vi "发送数据记录到文档(子VI).vi"(7 "错误输入":errorcluster, 9 "字符串":string="报文记录", 10 "数组":string[](array[string])) -> (0 "错误输出":errorcluster)   [LabVIEW 2022 SP3, in "工况数据上传.lvlib"]
panel:
  out "路径":path
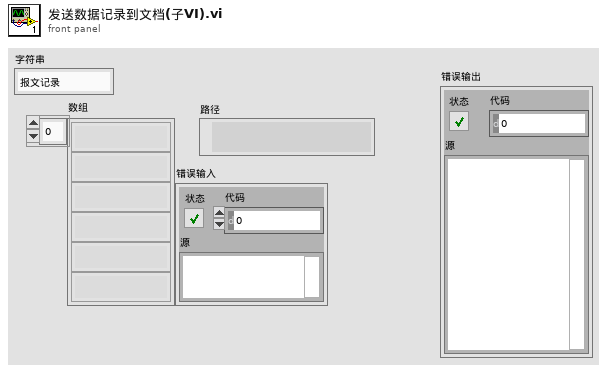
[diagram p1: front panel]
types:
  T1 = typedef "LVDateTimeRec.ctl" = cluster{"秒数的小数部分":dbl, "秒":i32, "分":i32, "时":i32, "日":i32, "月":i32, "年":i32, "天数（周）":i32, "天数（年）":i32, "DST":i32}
  T2 = enum16{"open", "replace", "create", "open or create", "replace or create", "replace or create with confirmation"}
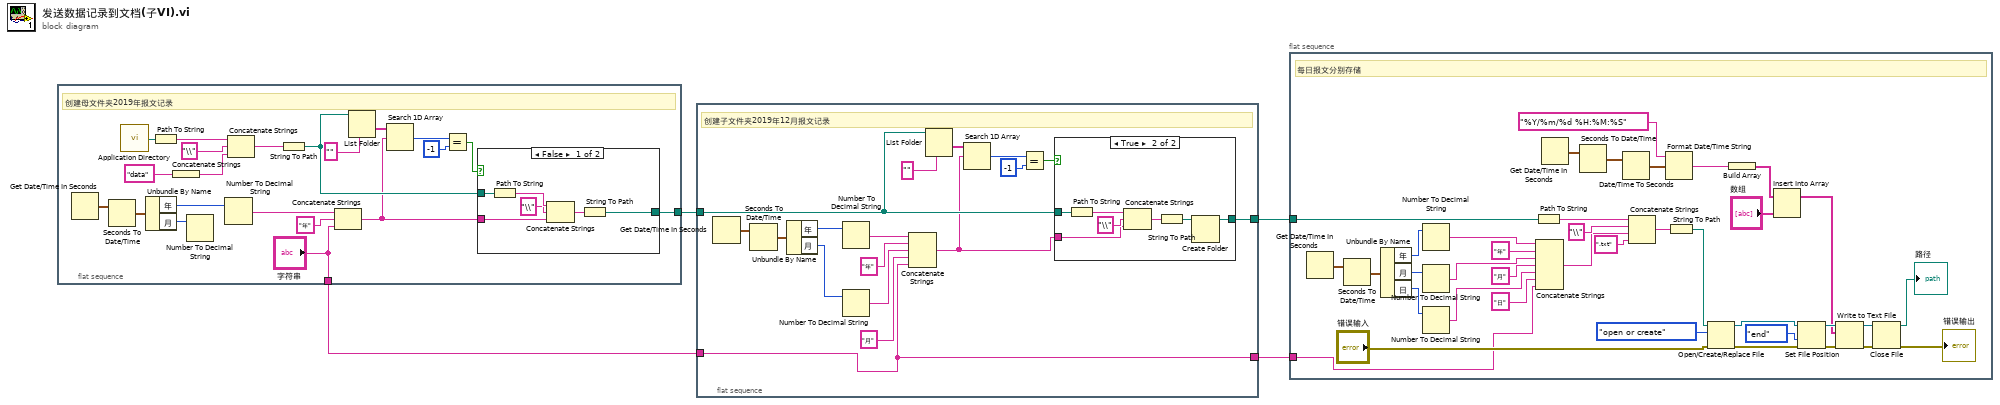
[diagram p0: block diagram]
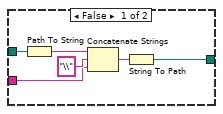
[diagram p2: hidden frame]
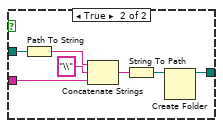
[diagram p3: hidden frame]
diagram:
  n1 = flat-sequence {
    tunnel: [w8] -> w4
    tunnel: ["字符串"] -> w2
    frame #0 {
      # "创建母文件夹2019年报文记录"
      n2 = Get Date/Time In Seconds() -> (seconds since 1Jan1904=w25:timestamp)
      n3 = Seconds To Date/Time(time stamp (now)=w25) -> (date time rec=w24:T1)  [unwired: 1 in]
      n4 = call <vilib>:"Application Directory.vi"() -> ("Application Directory"=w13:path)
      n5 = Unbundle By Name(w24) -> ("年"=w23:i32, "月"=w22:i32)
      n6 = Path To String(path=w13) -> (string=w16:string)
      n7 = Concatenate Strings("data" ("名称或相对路径")) -> (w5:string)
      n8 = Number To Decimal String(number=w22) -> ()  [unwired: 1 in, 1 out]
      n9 = Number To Decimal String(number=w23) -> (decimal integer string=w10:string)  [unwired: 1 in]
      n10 = Concatenate Strings(w16, "\\" ("字符串"), w5) -> (w14:string)
      n11 = String To Path(string=w14) -> (path=w12:path)
      n12 = Concatenate Strings(w10, "年" ("字符串"), "字符串") -> (w9:string)
      n13 = List Folder(path=w12, pattern="" ("类型")) -> (folder names=w17:string[])  [unwired: 2 in, 3 out]
      n14 = Search 1D Array(1D array=w17, element=w9) -> (index of element=w21:i32)  [unwired: 1 in]
      n15 = Equal?(x=w21, y=-1) -> (x = y?=w19:bool)
      n16 = case shown="False" w19 {
        tunnel: w12 -> [w29 w37]
        tunnel: w9 -> [w28 w34]
        tunnel: [w27 w38] -> w8
        frame False {
          n17 = Path To String(path=w29) -> (string=w31:string)
          n18 = Concatenate Strings(w31, "\\" ("字符串"), w28) -> (w26:string)
          n19 = String To Path(string=w26) -> (path=w27:path)
        }
        frame True {
          n20 = Path To String(path=w37) -> (string=w36:string)
          n21 = Concatenate Strings(w36, "\\" ("字符串"), w34) -> (w32:string)
          n22 = String To Path(string=w32) -> (path=w33:path)
          n23 = Create Folder(path (use dialog)=w33) -> (created path=w38:path)  [unwired: 2 in, 2 out]
        }
      }
    }
  }
  n24 = flat-sequence {
    tunnel: w4 -> [w42]
    tunnel: [w40] -> w3
    tunnel: w2 -> [w39]
    tunnel: [w39] -> w1
    frame #0 {
      # "创建子文件夹2019年12月报文记录"
      n25 = Get Date/Time In Seconds() -> (seconds since 1Jan1904=w45:timestamp)
      n26 = Seconds To Date/Time(time stamp (now)=w45) -> (date time rec=w46:T1)  [unwired: 1 in]
      n27 = Unbundle By Name(w46) -> ("年"=w47:i32, "月"=w48:i32)
      n28 = Number To Decimal String(number=w47) -> (decimal integer string=w50:string)  [unwired: 1 in]
      n29 = Number To Decimal String(number=w48) -> (decimal integer string=w44:string)  [unwired: 1 in]
      n30 = Concatenate Strings(w50, "年" ("字符串"), w44, "月" ("字符串"), w39) -> (w41:string)
      n31 = List Folder(path=w42, pattern="" ("类型")) -> (folder names=w55:string[])  [unwired: 2 in, 3 out]
      n32 = Search 1D Array(1D array=w55, element=w41) -> (index of element=w51:i32)  [unwired: 1 in]
      n33 = Equal?(x=w51, y=-1) -> (x = y?=w53:bool)
      n34 = case shown="True" w53 {
        tunnel: w42 -> [w58 w67]
        tunnel: w41 -> [w57 w64]
        tunnel: [w56 w68] -> w40
        frame False {
          n35 = Path To String(path=w58) -> (string=w61:string)
          n36 = Concatenate Strings(w61, "\\" ("字符串"), w57) -> (w59:string)
          n37 = String To Path(string=w59) -> (path=w56:path)
        }
        frame True {
          n38 = Path To String(path=w67) -> (string=w66:string)
          n39 = Concatenate Strings(w66, "\\" ("字符串"), w64) -> (w63:string)
          n40 = String To Path(string=w63) -> (path=w62:path)
          n41 = Create Folder(path (use dialog)=w62) -> (created path=w68:path)  [unwired: 2 in, 2 out]
        }
      }
    }
  }
  n42 = flat-sequence {
    tunnel: w3 -> [w80]
    tunnel: w1 -> [w69]
    frame #0 {
      # "每日报文分别存储"
      n43 = Get Date/Time In Seconds() -> (seconds since 1Jan1904=w104:timestamp)
      n44 = Seconds To Date/Time(time stamp (now)=w104) -> (date time rec=w103:T1)  [unwired: 1 in]
      n45 = Unbundle By Name(w103) -> ("年"=w102:i32, "月"=w101:i32, "日"=w98:i32)
      n46 = Number To Decimal String(number=w102) -> (decimal integer string=w99:string)  [unwired: 1 in]
      n47 = Number To Decimal String(number=w101) -> (decimal integer string=w105:string)  [unwired: 1 in]
      n48 = Number To Decimal String(number=w98) -> (decimal integer string=w96:string)  [unwired: 1 in]
      n49 = Path To String(path=w80) -> (string=w88:string)
      n50 = Concatenate Strings(w99, "年" ("字符串"), w105, "月" ("字符串"), w96, "日" ("字符串"), w69) -> (w82:string)
      n51 = Get Date/Time In Seconds() -> (seconds since 1Jan1904=w72:timestamp)
      n52 = Seconds To Date/Time(time stamp (now)=w72) -> (date time rec=w75:T1)  [unwired: 1 in]
      n53 = Date/Time To Seconds(2:w75) -> (0:w73:timestamp)  [unwired: 1 in]
      n54 = Concatenate Strings(w88, "\\" ("字符串"), w82, ".txt" ("字符串")) -> (w90:string)
      n55 = Format Date/Time String(time format string (%c)="%Y/%m/%d %H:%M:%S" ("时间格式字符串(%c)"), seconds (now)=w73) -> (date/time string=w76:string)  [unwired: 1 in]
      n56 = String To Path(string=w90) -> (path=w86:path)
      n57 = Open/Create/Replace File(file path (use dialog)=w86, error in="错误输入", operation (0:open)=T2."open or create" ("操作(0:open)")) -> (refnum out=w91:refnum<file>, error out=w92:errorcluster)  [unwired: 3 in, 1 out]
      n58 = Build Array(w76) -> (w71:string[])
      n59 = Insert Into Array(array=w71, new element="数组") -> (w70:string[])  [unwired: 1 in]
      n60 = Set File Position(refnum=w91, from (0:start)=enum16{"start", "end", "current"}."end" ("自（0:起始）"), error in=w92) -> (refnum out=w93:refnum<file>, error out=w94:errorcluster)  [unwired: 1 in]
      n61 = Write to Text File(file (use dialog)=w93, text=w70, error in=w94) -> (refnum out=w85:refnum<file>, error out=w84:errorcluster)  [unwired: 1 in, 1 out]
      n62 = Close File(refnum=w85, error in=w84) -> (path=→"路径":path, error out=→"错误输出":errorcluster)
    }
  }
